vi "Transform.vi"(7 "Type X":T2(ring), 8 "error in (no error)":errorcluster caption="entrée d'erreur (pas d'erreur)", 9 "y":string[][](array[string]), 10 "X":string[][](array[string]), 11 "AdditiveChi2Sampler.lvclass":refnum<class "AdditiveChi2Sampler.lvclass">) -> (0 "error out":errorcluster caption="sortie d'erreur", 2 "Data":T1, 3 "AdditiveChi2Sampler.lvclass":refnum<class "AdditiveChi2Sampler.lvclass">)   [LabVIEW 2020, in "AdditiveChi2Sampler.lvclass"]
doc: "Apply approximate feature map to X.\n\nReturns : \n\n- X_new : {array, sparse matrix}, shape = (n_samples, n_features * (2*sample_steps + 1))\nWhether the return value is an array of sparse matrix depends on the type of the input X."
uses:
  AdditiveChi2Sampler.lvclass
  AdditiveChi2Sampler.lvclass/AdditiveChi2Sampler.ctl
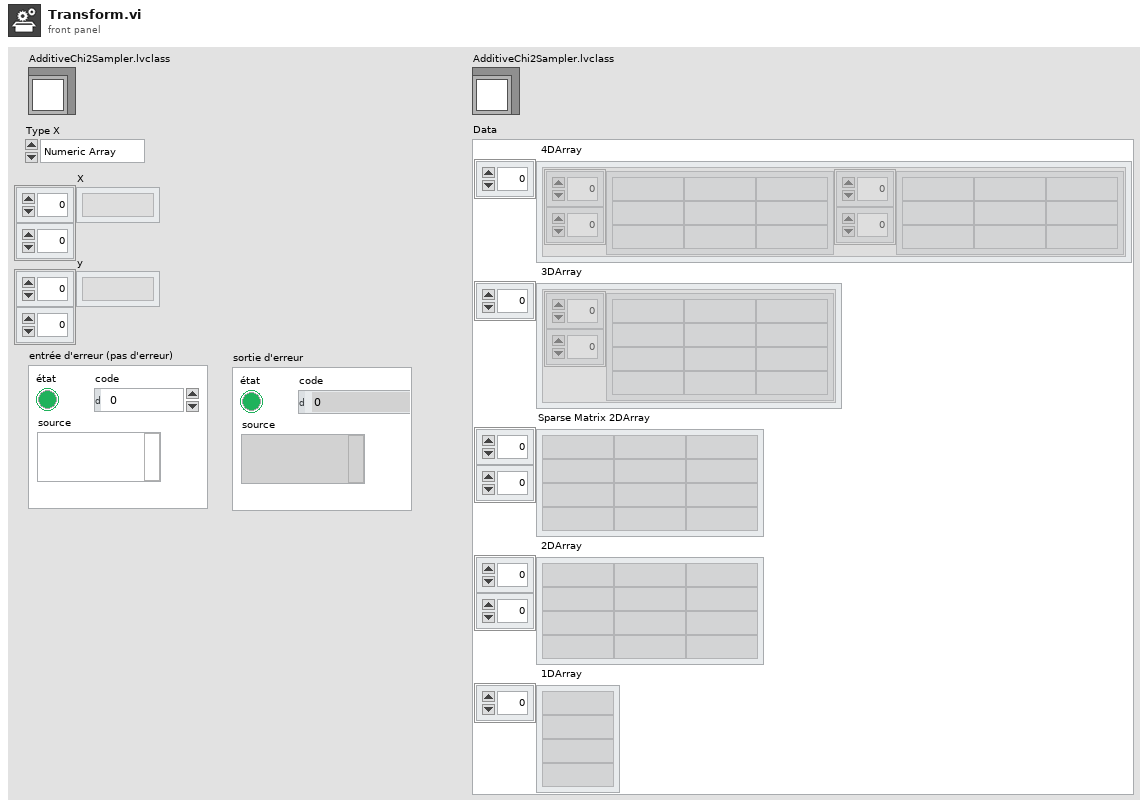
[diagram p1: front panel]
types:
  T1 = cluster{" 4DArray":cluster{"1":string[][], "2":string[][]}[], " 3DArray":cluster{"Tableau":string[][]}[], "Sparse Matrix 2DArray":string[][], " 2DArray":string[][], " 1DArray":string[]}
  T2 = enum16{"Numeric Array", "String Array", "Sparse"}
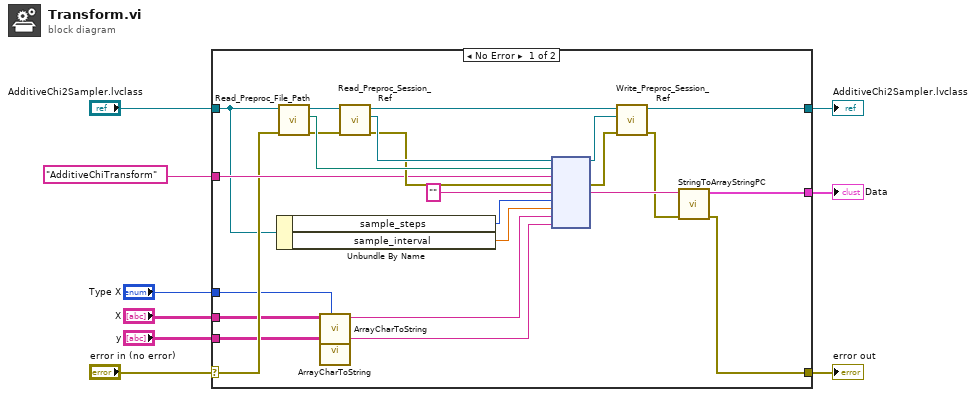
[diagram p0: block diagram]
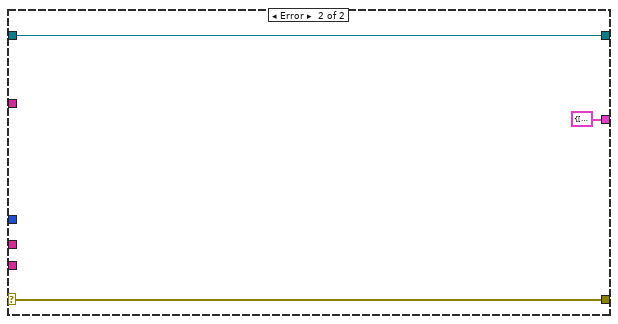
[diagram p2: hidden frame]
diagram:
  n1 = case shown="No Error" "error in (no error)" {
    selector: "error in (no error)" -> [w21 w36]
    tunnel: [w10 w36] -> w8
    tunnel: [w14 w35] -> w6
    tunnel: "AdditiveChi2Sampler.lvclass" -> [w20 w35]
    tunnel: "AdditiveChiTransform" ("Fonction") -> [w22 _]
    tunnel: "X" -> [w19 _]
    tunnel: "y" -> [w17 _]
    tunnel: "Type X" -> [w18 _]
    tunnel: [w11 T1 {" 4DArray"=[], " 3DArray"=[], "Sparse Matrix 2DArray"=[], " 2DArray"=[], " 1DArray"=[]} ("Data")] -> w1
    frame No Error {
      n2 = Unbundle By Name(w20) -> ("sample_steps"=w24:i32, "sample_interval"=w23:dbl)
      n3 = call-dynamic "Read_Preproc_File_Path.vi"("error in (no error)"=w21, "Python in"=w20) -> ("error out"=w28:errorcluster, "File_Path"=w31:path, "Python out"=w33:refnum<class "AdditiveChi2Sampler.lvclass">)  [unwired: 7 in]
      n4 = call "ArrayCharToString.vi"("Type"=w18, "TAB"=w19) -> ("Instruction"=w16:string)  [unwired: 9 in]
      n5 = call "ArrayCharToString.vi"("TAB"=w17) -> ("Instruction"=w15:string)  [unwired: 10 in]
      n6 = call-dynamic "Read_Preproc_Session_Ref.vi"("error in (no error)"=w28, "Python in"=w33) -> ("error out"=w29:errorcluster, "Session_ref"=w30:refnum<k35>, "Python out"=w32:refnum<class "AdditiveChi2Sampler.lvclass">)  [unwired: 7 in]
      n7 = node(w30, w31, w22, w29, "", w24, w23, w16, w15) -> (w25:refnum<k35>, w27:errorcluster, w13:string)  [unwired: 4 in, 2 out]
      n8 = call-dynamic "Write_Preproc_Session_Ref.vi"("error in (no error)"=w27, "Session_ref"=w25, "Python in"=w32) -> ("error out"=w12:errorcluster, "Python out"=w14:refnum<class "AdditiveChi2Sampler.lvclass">)  [unwired: 7 in]
      n9 = call "StringToArrayStringPC.vi"("sortie d'erreur"=w12, "Return value"=w13) -> ("sortie d'erreur"=w10:errorcluster, "Data"=w11:T1)  [unwired: 8 in]
    }
    frame Error {
    }
  }
  "error out" <- w8
  "AdditiveChi2Sampler.lvclass" <- w6
  "Data" <- w1
